vi "Create New UserEvents Handler.vi"(7 "Handler.UserEvent in":refnum<class "Handler.UserEvent.lvclass">, 8 "error in (no error)":errorcluster, 10 "Name":string, 11 "Level":T1(ring)) -> (0 "error out":errorcluster, 3 "Handler.UserEvent out":refnum<class "Handler.UserEvent.lvclass">)   [LabVIEW 2017, in "Error Log.lvlib" / "Handler.UserEvent.lvclass"]
uses:
  Handler.UserEvent.lvclass
  \\192.168.1.40\Neosoft/Partage/Dossiers Personnels/BRO/DevTools_BR/wc/ErrorLog/src/Handler/Handler.lvclass
  Handler/Handler.lvclass
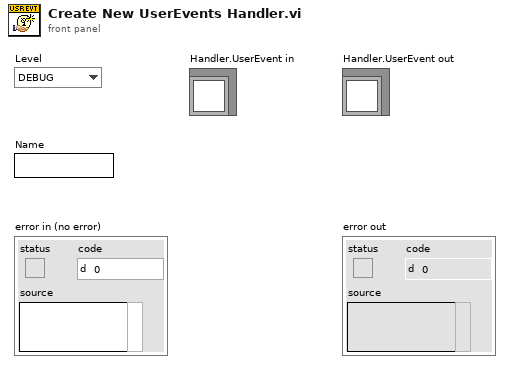
[diagram p1: front panel]
types:
  T1 = enum16{"DEBUG", "INFO", "WARNING", "ERROR", "CRITICAL"}
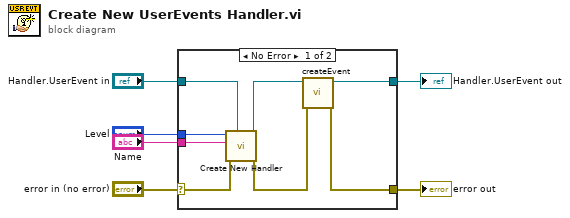
[diagram p0: block diagram]
diagram:
  n1 = case shown="No Error" "error in (no error)" {
    selector: "error in (no error)" -> [w13 w16]
    tunnel: [w9 w16] -> w5
    tunnel: [w11 w15] -> w3
    tunnel: "Handler.UserEvent in" -> [w14 w15]
    tunnel: "Level" -> [w8 _]
    tunnel: "Name" -> [w7 _]
    frame No Error {
      n2 = call "Create New Handler.vi"("Handler type"=w14, "error in (no error)"=w13, "Name"=w7, "Level"=w8) -> ("error out"=w10:errorcluster, "Handler"=w12:refnum<class "Handler.UserEvent.lvclass">)  [unwired: 6 in]
      n3 = call-dynamic "createEvent.vi"("error in (no error)"=w10, "Handler.UserEvent in"=w12) -> ("error out"=w9:errorcluster, "Handler.UserEvent out"=w11:refnum<class "Handler.UserEvent.lvclass">)  [unwired: 8 in]
    }
    frame Error {
    }
  }
  "error out" <- w5
  "Handler.UserEvent out" <- w3
